vi "ief_reset_axis_measuring_mode.vi"(2 "error in (no error)":errorcluster, 3 "Axis Number":u16=1 min=1 max=16, 4 "Tagprefix in":refnum<k21>) -> (0 "error out (no error)":errorcluster, 1 "Tagprefix out":refnum<k21>)   [LabVIEW 2015, in "IEF Werner.lvlib"]
doc: "The VI deactivates the measuring mode of the chosen axis.\n\nPA-Control EP:\n- the motor regains power\n- brakes are deactivated\n- synchronisation of the roatary encoder is performed\n- axis position is adopted from rotary encoder\n- supervisory of rotary encoder and power supply standby are activated\n\nAxis Number Range:\n01, 10 hex\n1, 16 dec"
uses:
  IEF Werner.lvlib
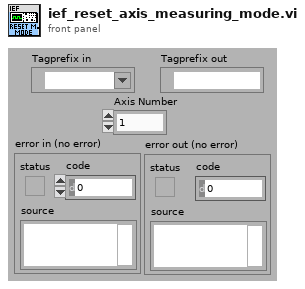
[diagram p1: front panel]
types:
  T1 = typedef "Semaphore RefNum" = refnum<k1>
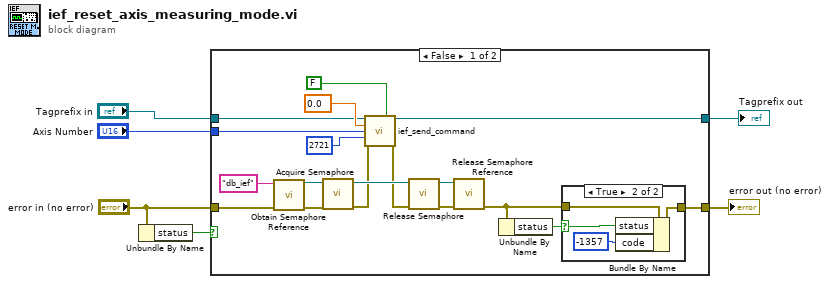
[diagram p0: block diagram]
diagram:
  n1 = Unbundle By Name("error in (no error)") -> ("status"=w3:bool)
  n2 = case shown="False" w3 {
    tunnel: "Axis Number" -> [w22 _]
    tunnel: "error in (no error)" -> [w14 w31]
    tunnel: [w21 w31] -> w5
    tunnel: "Tagprefix in" -> [w8 w30]
    tunnel: [w7 w30] -> w1
    frame False {
      n3 = call <vilib>:"Obtain Semaphore Reference.vi"("error in (no error)"=w14, "name (unnamed)"="db_ief") -> ("error out"=w18:errorcluster, "semaphore"=w19:T1)  [unwired: 3 in, 1 out]
      n4 = call <vilib>:"Acquire Semaphore.vi"("error in (no error)"=w18, "semaphore"=w19) -> ("error out"=w13:errorcluster, "semaphore out"=w17:T1)  [unwired: 3 in, 1 out]
      n5 = call "ief_send_command.vi"("Tagprefix in"=w8, "Command datum of type real"=FALSE, "Command datum"=sgl 0.0, "Command parameter"=w22, "Command code"=u16 2721, "error in (no error)"=w13) -> ("Tagprefix out"=w7:refnum<k21>, "error out (no error)"=w11:errorcluster)  [unwired: 4 in, 4 out]
      n6 = call <vilib>:"Release Semaphore.vi"("error in (no error)"=w11, "semaphore"=w17) -> ("error out"=w16:errorcluster, "semaphore out"=w15:T1)  [unwired: 4 in]
      n7 = call <vilib>:"Release Semaphore Reference.vi"("error in (no error)"=w16, "semaphore"=w15) -> ("error out"=w12:errorcluster)  [unwired: 8 in, 1 out]
      n8 = Unbundle By Name(w12) -> ("status"=w10:bool)
      n9 = case shown="True" w10 {
        selector: w10 -> [_ w26]
        tunnel: [w25 w28] -> w21
        tunnel: w12 -> [w25 w29]
        frame False {
        }
        frame True {
          n10 = Bundle By Name(cluster=w29, "status"=w26, "code"=-1357) -> (w28:errorcluster)
        }
      }
    }
    frame True {
    }
  }
  "error out (no error)" <- w5
  "Tagprefix out" <- w1
